vi "Translation3d_UnaryMinus.vi"(11 "In Translation3d":T1 {"Z" format="%14.3f"; "Y" format="%14.3f"; "X" format="%14.3f"}) -> (3 "Out Translation3d":T1 {"Z" format="%14.3f"; "Y" format="%14.3f"; "X" format="%14.3f"})   [LabVIEW 2019, in "Trajectory_Library.lvlib"]
doc: "Returns the inverse of the current translation. This is equivalent to rotating by 180 degrees, flipping the point over both axes, or simply negating both components of the translation.\n \nParameters:\n - In Translation - This translation data structure\n\nResult:\n - Out Translation - The inverse of the current translation."
uses:
  Trajectory_Library.lvlib
  TRANSLATION3D.ctl
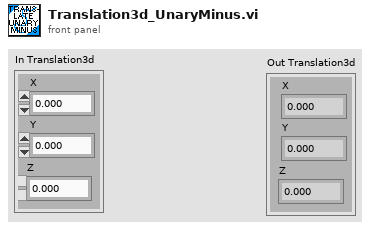
[diagram p1: front panel]
types:
  T1 = typedef "Trajectory_Library.lvlib/TRANSLATION3D.ctl" = cluster{"X":dbl, "Y":dbl, "Z":dbl}
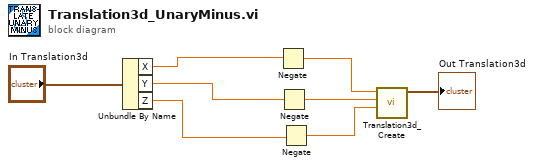
[diagram p0: block diagram]
diagram:
  n1 = Unbundle By Name("In Translation3d") -> ("X"=w6:dbl, "Y"=w4:dbl, "Z"=w1:dbl)
  n2 = Negate(x=w6) -> (-x=w5:dbl)
  n3 = Negate(x=w4) -> (-x=w3:dbl)
  n4 = Negate(x=w1) -> (-x=w2:dbl)
  n5 = call "Translation3d_Create.vi"("Z"=w2, "Y"=w3, "X"=w5) -> ("TRANSLATION3D"=→"Out Translation3d":T1)  [unwired: 8 in]
